vi "Dynamic To Waveform.vi"(4 "Input":dynamicdata(waveform), 5 "index":i32) -> (1 "Output":waveform(dbl))   [LabVIEW 2020]
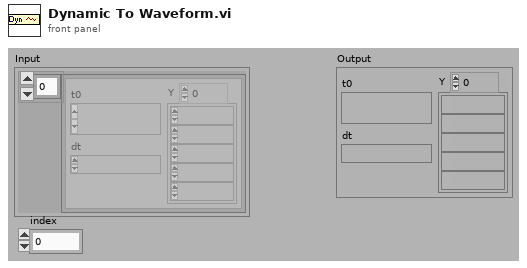
[diagram p1: front panel]
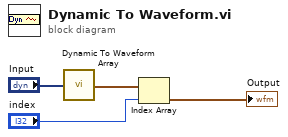
[diagram p0: block diagram]
diagram:
  n1 = call <vilib>:"Dynamic To Waveform Array.vi"("Input"="Input") -> ("Output"=w3:waveform(dbl)[])  [unwired: 4 in]
  n2 = Index Array(array=w3, index="index") -> (element=→"Output":waveform(dbl))
